vi "ActionVIOnDelete.vi"(6 "All deleted Refs":T1[](array[typedef]) format="%.0x", 8 "error in (no error)":errorcluster, 11 "Item Ref in":T1 format="%.0x") -> (0 "error out":errorcluster, 3 "Item Ref out":T1 format="%.0x")   [LabVIEW 2016, in "FPGA RM System Definition API.lvlib"]
uses:
  FPGA RM System Definition API.lvlib
  <vilib>/NI Veristand/Custom Device API/Custom Device Item Ref.ctl
  <vilib>/NI VeriStand/Custom Device API/Custom Device API.lvlib
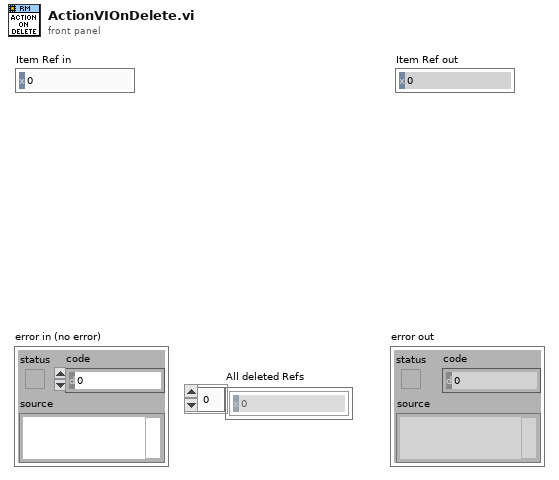
[diagram p1: front panel]
types:
  T1 = typedef "Custom Device API.lvlib/Custom Device Item Ref.ctl" = u64
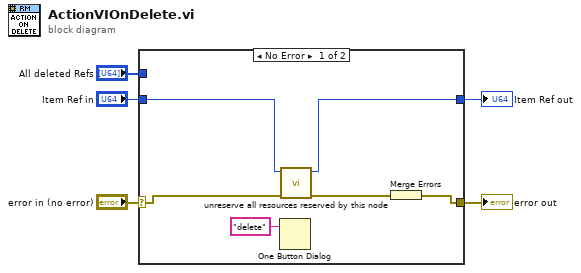
[diagram p0: block diagram]
diagram:
  n1 = case shown="No Error" "error in (no error)" {
    selector: "error in (no error)" -> [w9 w13]
    tunnel: [w10 w13] -> w4
    tunnel: "Item Ref in" -> [w8 w12]
    tunnel: [w7 w12] -> w2
    tunnel: "All deleted Refs" -> [_ _]
    frame No Error {
      n2 = One Button Dialog(message="delete") -> ()  [unwired: 1 in, 1 out]
      n3 = call "unreserve all resources reserved by this node.vi"("error in (no error)"=w9, "Item Ref in"=w8) -> ("error out"=w11:errorcluster, "Item Ref out"=w7:T1)  [unwired: 8 in]
      n4 = Merge Errors(w11) -> (w10:errorcluster)
    }
    frame Error {
    }
  }
  "error out" <- w4
  "Item Ref out" <- w2
